vi "fgv_main-q.vi"(7 "cmd":enum16{"ini", "read", "write", "close"}(ring), 8 "error in":errorcluster, 11 "menu":T1) -> (0 "error out":errorcluster, 3 "queue out":refnum<queue>)   [LabVIEW 2019]
uses:
  _ctrl/menu_main.ctl
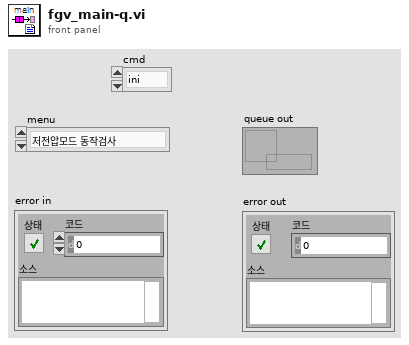
[diagram p1: front panel]
types:
  T1 = typedef "menu_main.ctl" = enum16{"저전압모드 동작검사", "저전압모드 접촉저항", "고전압모드 동작검사"}
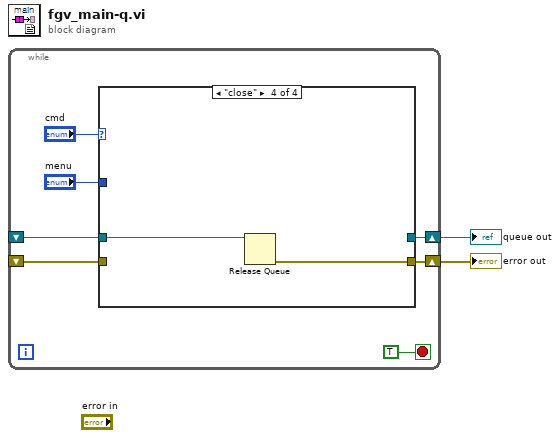
[diagram p0: block diagram]
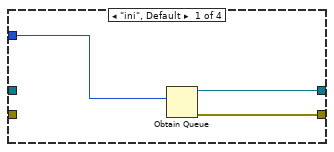
[diagram p2: hidden frame]
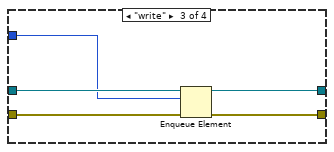
[diagram p4: hidden frame]
diagram:
  n1 = while {
    shift-right: [w7] -> w2
    shift-left: _ -> [w4]
    shift-right: [w6] -> w1
    shift-left: _ -> [w3]
    stop <- TRUE stop-if-true
    n2 = case shown="\"close\"" "cmd" {
      tunnel: [w12 w14 w16 _] -> w7
      tunnel: [w11 w13 w17 w21] -> w6
      tunnel: "menu" -> [w10 _ w15 _]
      tunnel: w4 -> [_ w14 w19 w20]
      tunnel: w3 -> [_ w13 w18 _]
      frame "ini", Default {
        n3 = Obtain Queue(element data type=w10) -> (queue out=w12:refnum<queue>, error out=w11:errorcluster)  [unwired: 4 in, 1 out]
      }
      frame "read" {
      }
      frame "write" {
        n4 = Enqueue Element(queue=w19, element=w15, error in (no error)=w18) -> (queue out=w16:refnum<queue>, error out=w17:errorcluster)  [unwired: 1 in, 1 out]
      }
      frame "close" {
        n5 = Release Queue(queue=w20) -> (error out=w21:errorcluster)  [unwired: 2 in, 2 out]
      }
    }
  }
  "queue out" <- w2
  "error out" <- w1
